vi "ReadSetpointTemp.vi"() -> (2 "error out":errorcluster, 3 "Probe 1 temperature":dbl format="%.2f")   [LabVIEW 2009]
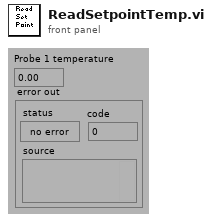
[diagram p1: front panel]
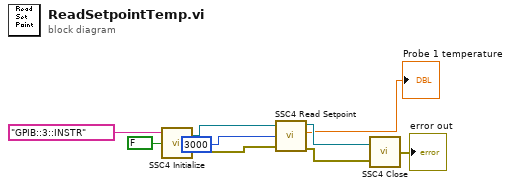
[diagram p0: block diagram]
diagram:
  n1 = call "SSC4 Initialize.vi"("reset"=FALSE, "instrument descriptor"="GPIB::3::INSTR") -> ("error out"=w3:errorcluster, "VISA session"=w4:refnum<visa-resource-name>)  [unwired: 1 in]
  n2 = call "SSC4 Read Setpoint.vi"("error in (no error)"=w3, "Command Delay (ms)"=u32 3000, "Visa Session"=w4) -> ("error out"=w5:errorcluster, "Current Setpoint"=→"Probe 1 temperature":dbl, "Dup Visa Session"=w6:refnum<visa-resource-name>)  [unwired: 2 in, 1 out]
  n3 = call "SSC4 Close.vi"("error in (no error)"=w5, "VISA session"=w6) -> ("error out"=→"error out":errorcluster)
